vi "氨氮 interface.vi"   [LabVIEW 2016, in "MB SLAVE.lvlib"]
uses:
  MB SLAVE.lvlib
types:
  T1 = typedef "氨氮交互.ctl" = cluster{"状态告警区":cluster{"系统时间":timestamp, "工作状态":u16, "测量模式":enum16{"待机", "连续模式", "周期模式", "定点模式", "受控模式", "手动模式"}, "告警代码":u16, "故障代码":u16, "日志代码":u16, "软件版本":u16, "F0":sgl, "F1":sgl, "F2":sgl, "F3":sgl, "T":sgl, "H":sgl, "id":u16, "flowid":u16, "量程":u16, "总磷控温温度1":sgl, "营养盐控温温度2":sgl, "ADC":sgl}, "平台试剂余量百分比":sgl, "关键参数":cluster{"测量量程":dbl, "测量精度":dbl, "测量间隔":dbl, "消解温度":dbl, "消解时长":dbl, "空白校准时间":timestamp, "曲线截距":dbl, "曲线斜率":dbl, "测量检出限":dbl, "测量信号值":dbl, "线性相关系数":dbl, "二次多项式系数":dbl, "标样校准时间":timestamp, "稀释倍数":dbl, "三项式系数":dbl, "空白标定系数":dbl, "量程系数":dbl, "F0/ORPA":dbl, "F1/ORPB":dbl, "F2/ORPK":dbl, "F3":dbl, "F4":dbl, "F5":dbl, "F6":dbl, "F7":dbl, "X0/滴定数":dbl, "量程":dbl}, "关键参数改变":bool, "校准信息":cluster{"低标液1浓度":dbl, "低标液1信号值":dbl, "低标液1启用":u16, "低标液2浓度":dbl, "低标液2信号值":dbl, "低标液2启用":u16, "低标液3浓度":dbl, "低标液3信号值":dbl, "低标液3启用":u16, "低标液4浓度":dbl, "低标液4信号值":dbl, "低标液4启用":u16, "低标液5浓度":dbl, "低标液5信号值":dbl, "低标液5启用":u16, "高标液1浓度":dbl, "高标液1信号值":dbl, "高标液1启用":u16, "高标液2浓度":dbl, "高标液2信号值":dbl, "高标液2启用":u16, "高标液3浓度":dbl, "高标液3信号值":dbl, "高标液3启用":u16, "高标液4浓度":dbl, "高标液4信号值":dbl, "高标液4启用":u16, "高标液5浓度":dbl, "高标液5信号值":dbl, "高标液5启用":u16, "低斜率":dbl, "低截距":dbl, "低二次多项式系数":dbl, "低线性相关系数":dbl, "高斜率":dbl, "高截距":dbl, "高二次多项式系数":dbl, "高线性相关系数":dbl}, "校准信息改变":bool}
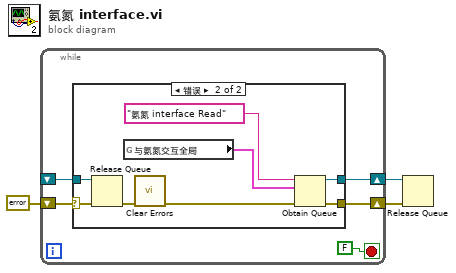
[diagram p0: block diagram]
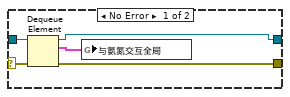
[diagram p2: hidden frame]
diagram:
  n1 = while {
    shift-right: [w8] -> w1
    shift-left: errorcluster {"status"=TRUE, "code"=0, "source"=""} ("error out") -> [w7]
    shift-right: [w6] -> w2
    shift-left: _ -> [w5]
    stop <- FALSE stop-if-true
    n2 = case shown="错误" w7 {
      selector: w7 -> [w12 w18]
      tunnel: [w10 w20] -> w8
      tunnel: [w11 w19] -> w6
      tunnel: w5 -> [w13 w17]
      frame No Error {
        n3 = Dequeue Element(queue=w13, error in (no error)=w12) -> (queue out=w11:refnum<queue>, element=w9:T1, error out=w10:errorcluster)  [unwired: 1 in, 1 out]
        n4 = global write "modbus slave全局.vi" "与氨氮交互全局"(w9) -> ()
      }
      frame Error {
        n5 = Release Queue(queue=w17, error in (no error)=w18) -> (error out=w16:errorcluster)  [unwired: 1 in, 2 out]
        n6 = global read "modbus slave全局.vi" "与氨氮交互全局"() -> (w14:T1)
        n7 = call <vilib>:"Clear Errors.vi"("error in (no error)"=w16) -> ("error out"=w15:errorcluster)  [unwired: 5 in, 1 out]
        n8 = Obtain Queue(name (unnamed)="氨氮 interface Read" ("写入方名称"), element data type=w14, error in (no error)=w15) -> (queue out=w19:refnum<queue>, error out=w20:errorcluster)  [unwired: 2 in, 1 out]
      }
    }
  }
  n9 = Release Queue(queue=w2, error in (no error)=w1) -> ()  [unwired: 1 in, 3 out]
